vi "DXFTest.vi"() -> ()   [LabVIEW 2020]
uses:
  C:/Projects/DXFViewer/LabviewDXFViewer/LabviewDXFViewer/bin/Debug/LabviewDXFViewer.exe
  LabviewDXFViewer/bin/Debug/LabviewDXFViewer.exe
panel:
  in  "DXFCanvas":refnum<k24>(container)
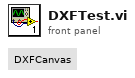
[diagram p1: front panel]
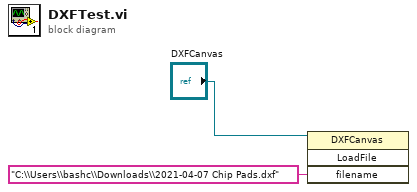
[diagram p0: block diagram]
diagram:
  n1 = invoke class="DXFCanvas" method="LoadFile"(reference="DXFCanvas", "filename"="C:\\Users\\bashc\\Downloads\\2021-04-07 Chip Pads.dxf") -> ()  [unwired: 2 in, 4 out]
